vi "Action.vi"(8 "error in (no error)":errorcluster, 10 "Actor in":refnum<class "Tamagotchi Basic Actor.lvclass">, 11 "Update UI Message in":refnum<class "Update UI Message.lvclass">) -> (0 "error out":errorcluster, 2 "Actor out":refnum<class "Tamagotchi Basic Actor.lvclass">, 3 "Update UI Message out":refnum<class "Update UI Message.lvclass">)   [LabVIEW 2026, in "Update UI Message.lvclass"]
uses:
  Update UI Message.lvclass
  Tamagotchi Basic Actor/Tamagotchi Basic Actor.lvclass
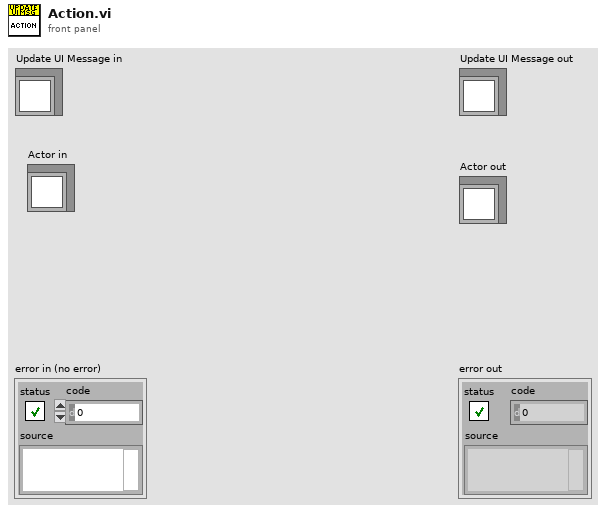
[diagram p1: front panel]
types:
  T1 = typedef "Controls Cluster.ctl" = cluster{"Pict Ring":refnum<vi>, "Mood":refnum<vi>, "Cleanliness":refnum<vi>, "Hunger":refnum<vi>, "Energy":refnum<vi>, "Age (cycles)":refnum<vi>}
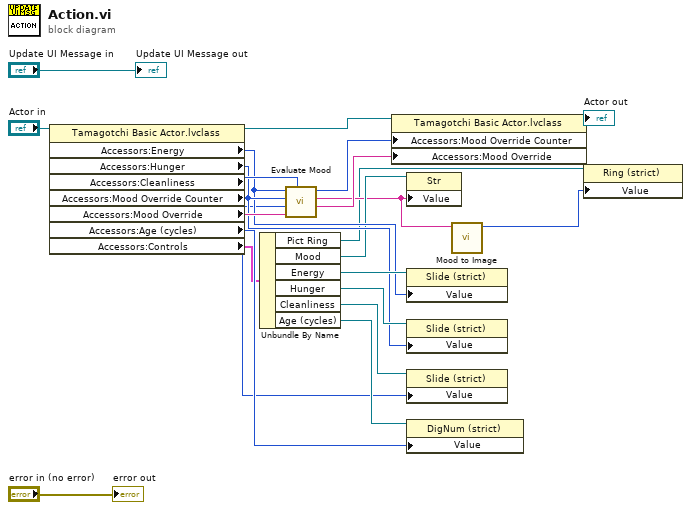
[diagram p0: block diagram]
diagram:
  n1 = property class="Tamagotchi Basic Actor.lvclass"(reference="Actor in") -> (reference out=w20:refnum<class "Tamagotchi Basic Actor.lvclass">, "Accessors:Energy"=w7:i16, "Accessors:Hunger"=w8:i16, "Accessors:Cleanliness"=w2:i16, "Accessors:Mood Override Counter"=w17:u32, "Accessors:Mood Override"=w16:string, "Accessors:Age (cycles)"=w12:u32, "Accessors:Controls"=w1:T1)  [unwired: 1 in, 1 out]
  n2 = Unbundle By Name(w1) -> ("Pict Ring"=w4:refnum<vi>, "Mood"=w6:refnum<vi>, "Energy"=w9:refnum<vi>, "Hunger"=w10:refnum<vi>, "Cleanliness"=w11:refnum<vi>, "Age (cycles)"=w13:refnum<vi>)
  n3 = call "Evaluate Mood.vi"("Mood Override Counter"=w17, "Override Mood"=w16, "Cleanliness"=w2, "Hunger"=w8, "Energy"=w7) -> ("Mood Override"=w15:string, "Mood"=w5:string, "Mood Override Counter out"=w18:u32)  [unwired: 4 in]
  n4 = property class="Tamagotchi Basic Actor.lvclass"(reference=w20, "Accessors:Mood Override Counter"=w18, "Accessors:Mood Override"=w15) -> (reference out=→"Actor out":refnum<class "Tamagotchi Basic Actor.lvclass">)  [unwired: 1 in, 1 out]
  n5 = property class="Str"(reference=w6, "Value"=w5) -> ()  [unwired: 1 in, 2 out]
  n6 = property class="Slide (strict)"(reference=w9, "Value"=w7) -> ()  [unwired: 1 in, 2 out]
  n7 = property class="Slide (strict)"(reference=w10, "Value"=w8) -> ()  [unwired: 1 in, 2 out]
  n8 = property class="Slide (strict)"(reference=w11, "Value"=w2) -> ()  [unwired: 1 in, 2 out]
  n9 = property class="DigNum (strict)"(reference=w13, "Value"=w12) -> ()  [unwired: 1 in, 2 out]
  n10 = call "Mood to Image.vi"("Mood"=w5) -> ("Image number"=w3:u16)  [unwired: 10 in]
  n11 = property class="Ring (strict)"(reference=w4, "Value"=w3) -> ()  [unwired: 1 in, 2 out]
  "error out" <- "error in (no error)"
  "Update UI Message out" <- "Update UI Message in"
